vi "AH read settings.vi"(8 "error in (no error)":errorcluster, 10 "Initial string":string, 11 "VISA Resource Name":refnum<visa-resource-name>) -> (0 "error out":errorcluster, 2 "Settings":string, 3 "VISA Resource Name Out":refnum<visa-resource-name>, 4 "Data titles":string[](array[string])=["Capacitance (F)", "Loss"])   [LabVIEW 2015]
uses:
  GPIB/VISA  Send Receive.vi
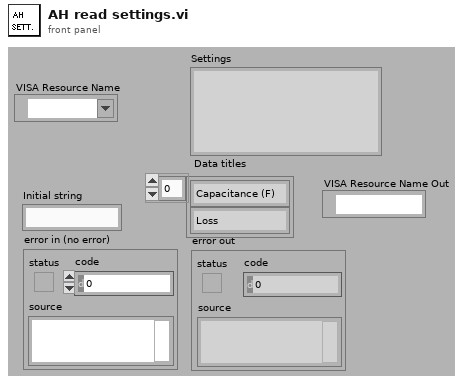
[diagram p1: front panel]
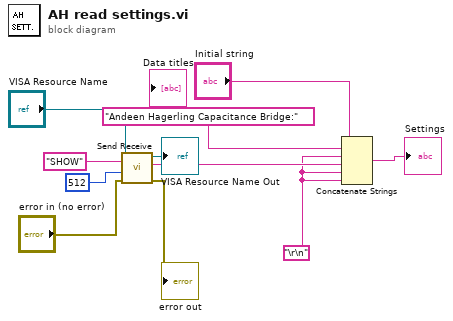
[diagram p0: block diagram]
diagram:
  w3 = "\r\n"
  n1 = call-poly "Send Receive.vi"("error in (no error)"="error in (no error)", "Receive count"=512 ("read count"), "data string in"="SHOW" ("write buffer"), "VISA Resource Name"="VISA Resource Name") -> ("error out"=→"error out":errorcluster, "data string out"=w7:string, "VISA Resource Name Out"=→"VISA Resource Name Out":refnum<visa-resource-name>)  [unwired: 5 in]
  n2 = Concatenate Strings("Initial string", "Andeen Hagerling Capacitance Bridge:" ("string"), w3, w7, w3, w3) -> (→"Settings":string)
